vi "Wait for Queue Termination.vi"(8 "error in (no error)":errorcluster, 11 "queue out":refnum<queue>) -> (0 "errorout":errorcluster)   [LabVIEW 2012, in "Command Queue.lvlib"]
uses:
  <vilib>/CommandQueue/Command Queue.lvlib
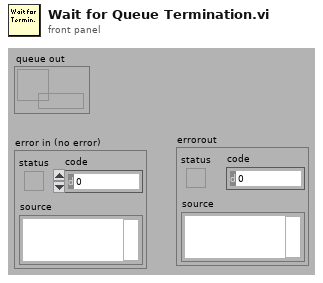
[diagram p1: front panel]
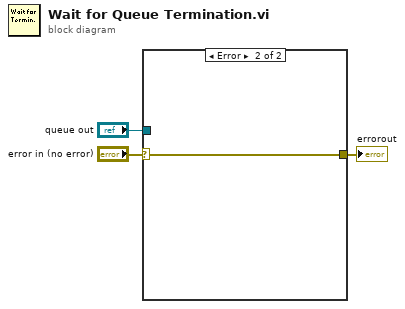
[diagram p0: block diagram]
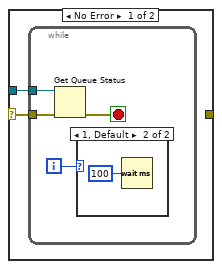
[diagram p2: hidden frame]
diagram:
  n1 = case shown="Error" "error in (no error)" {
    selector: "error in (no error)" -> [w4 w11]
    tunnel: "queue out" -> [w5 _]
    tunnel: [_ w11] -> w1
    frame No Error {
      n2 = while {
        tunnel: w5 -> [w9]
        tunnel: w4 -> [w7]
        i -> [w6]
        stop <- w8 stop-if-true
        n3 = Get Queue Status(queue=w9, error in (no error)=w7) -> (error out=w8:errorcluster)  [unwired: 1 in, 7 out]
        n4 = case shown="1, Default" w6 {
          frame 0 {
          }
          frame 1, Default {
            n5 = Wait (ms)(milliseconds to wait=u32 100) -> ()  [unwired: 1 out]
          }
        }
      }
    }
    frame Error {
    }
  }
  "errorout" <- w1
